vi "SIM921_check_Queue.vi"(8 "error in (no error)":errorcluster caption="Fehler (Eingang, kein Fehler)", 11 "queue":refnum<queue>) -> (0 "error out":errorcluster caption="Fehler (Ausgang)", 1 "SIM921-Control":T1, 3 "New Entries ?":bool)   [LabVIEW 2019]
uses:
  SIM921/SIM921_control_cluster.ctl
panel:
  out "Numerisches Anzeigeelement":i32
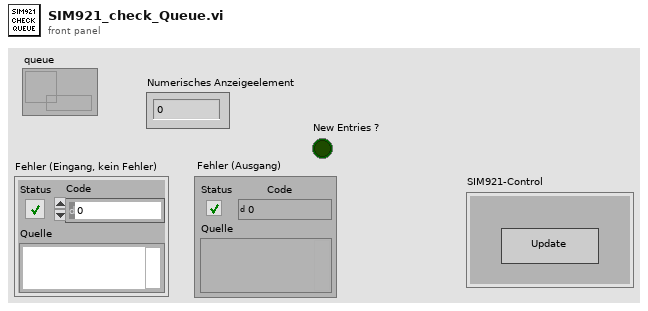
[diagram p1: front panel]
types:
  T1 = typedef "SIM921_control_cluster.ctl" = cluster{"Update":bool}
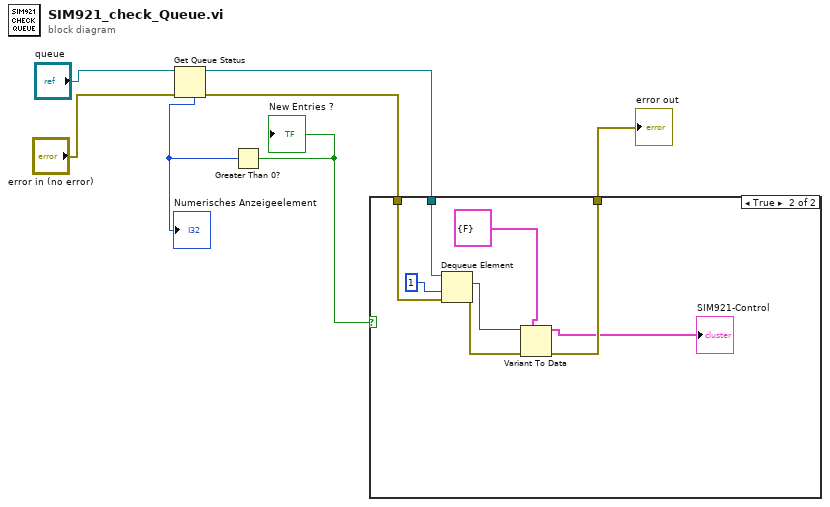
[diagram p0: block diagram]
diagram:
  n1 = Get Queue Status(queue="queue", error in (no error)="error in (no error)") -> (queue out=w3:refnum<queue>, error out=w2:errorcluster, # elements in queue=w5:i32)  [unwired: 1 in, 5 out]
  "Numerisches Anzeigeelement" <- w5
  n2 = Greater Than 0?(x=w5) -> (x > 0?=w4:bool)
  "New Entries ?" <- w4
  n3 = case shown="True" w4 {
    tunnel: w3 -> [_ w15]
    tunnel: w2 -> [w8 w16]
    tunnel: [w8 w11] -> w1
    frame False {
    }
    frame True {
      n4 = Dequeue Element(queue=w15, timeout in ms (-1)=1, error in (no error)=w16) -> (element=w13:variant, error out=w12:errorcluster)  [unwired: 2 out]
      n5 = Variant To Data(error in=w12, type=T1 {"Update"=FALSE} ("SIM921-Control"), Variant=w13) -> (data=→"SIM921-Control":T1, error out=w11:errorcluster)
    }
  }
  "error out" <- w1
